vi "WaveformCHart.vi"() -> ()   [LabVIEW 2022 SP3]
panel:
  out "Waveform Chart 2":dbl(graph)
  out "Waveform Graph":dbl[][](graph)
  in  "stop":bool
  out "Waveform Chart":dbl[](graph)
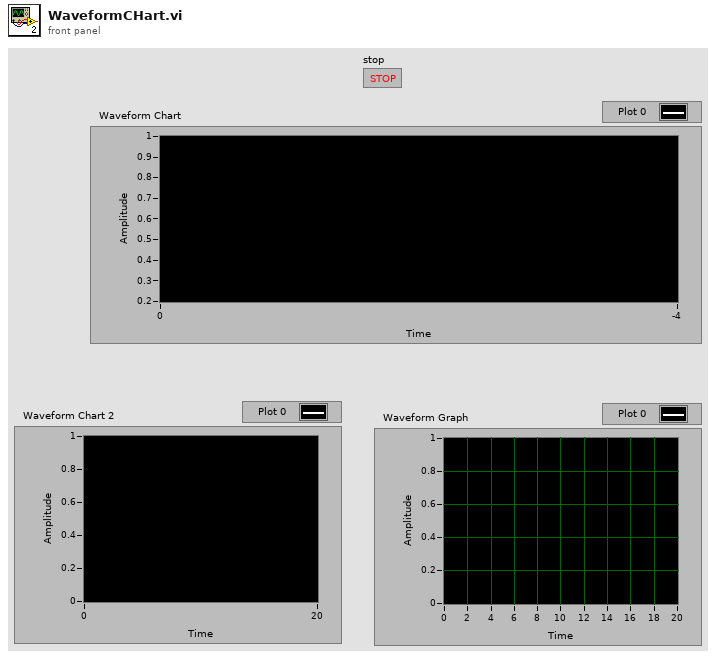
[diagram p1: front panel]
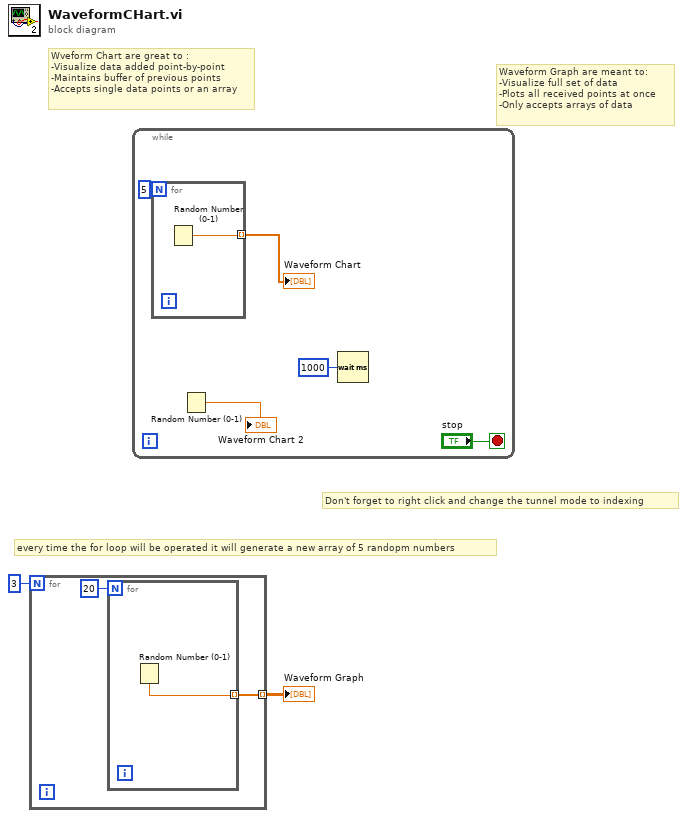
[diagram p0: block diagram]
diagram:
  # "Waveform Graph are meant to:\n-Visualize full set of data\n-Plots all received points at once \n-Only accepts arrays of data"
  # "Wveform Chart are great to :\n-Visualize data added point-by-point\n-Maintains buffer of previous points\n-Accepts single data points or an array"
  # "Don't forget to right click and change the tunnel mode to indexing"
  # "every time the for loop will be operated it will generate a new array of 5 randopm numbers"
  n1 = for {
    N: 3 -> [_]
    tunnel: [w3] -> w2 mode=indexing
    n2 = for {
      N: 20 -> [_]
      tunnel: [w5] -> w3 mode=indexing
      n3 = Random Number (0-1)() -> (number: 0 to 1=w5:dbl)
    }
  }
  "Waveform Graph" <- w2
  n4 = while {
    stop <- "stop" stop-if-true
    n5 = for {
      N: 5 -> [_]
      tunnel: [w11] -> w7 mode=indexing
      n6 = Random Number (0-1)() -> (number: 0 to 1=w11:dbl)
    }
    "Waveform Chart" <- w7
    n7 = Random Number (0-1)() -> (number: 0 to 1=→"Waveform Chart 2":dbl)
    n8 = Wait (ms)(milliseconds to wait=u32 1000) -> ()  [unwired: 1 out]
  }
